vi "Inicio_TurbiIN.vi"(0 "task/channels in":refnum<k21>="Turbi_IN", 5 "error in":errorcluster) -> (14 "Refnum out":refnum<k21>, 19 "error out":errorcluster)   [LabVIEW 2013]
uses:
  <vilib>/DAQmx/configure/timing.llb/DAQmx Timing (Sample Clock).vi
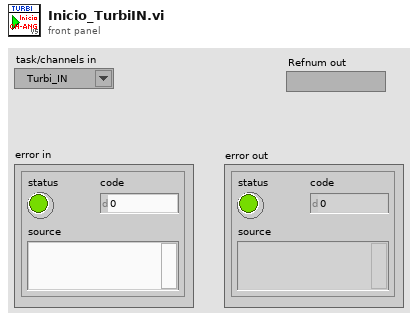
[diagram p1: front panel]
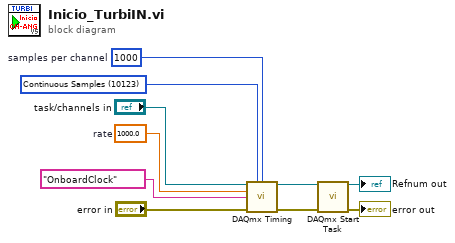
[diagram p0: block diagram]
diagram:
  w3 = 1000.0  # rate
  w2 = 1000  # samples per channel
  w1 = 10123 items=["Finite Samples"=10178, "Continuous Samples"=10123, "Hardware Timed Single Point"=12522] ("sample mode")
  n1 = call-poly <vilib>:"DAQmx Timing.vi"("task/channels in"="task/channels in", "sample mode"=w1, "samples per channel"=w2, "rate"=w3, "source"=tag "OnboardClock", "error in"="error in") -> ("task out"=w6:refnum<k21>, "error out"=w5:errorcluster)  [unwired: 8 in]
  n2 = call <vilib>:"DAQmx Start Task.vi"("task/channels in"=w6, "error in"=w5) -> ("task out"=→"Refnum out":refnum<k21>, "error out"=→"error out":errorcluster)  [unwired: 12 in]
